vi "Climb_Set.vi"   [LabVIEW 2019]
uses:
  Globals/Climb_Globals.vi
types:
  T1 = enum16{"No-Op", "Extending", "Clamping", "Balancing", "Manual_Control"}
  T2 = typedef "Climb_Cluster.ctl" = cluster{"Control_State":T3, "Extend_Climber?":bool, "Clamp?":bool, "Balance?":bool, "Transverse_Throttle":dbl, "Elevator_Throttle":dbl, "Control_Panel_Setpoint?":bool, "Auto-Balance":bool, "Pivot_Throttle":dbl}
  T3 = typedef "Climb_States.ctl" = enum16{"No-Op", "Extending", "Clamping", "Balancing", "Manual_Control"}
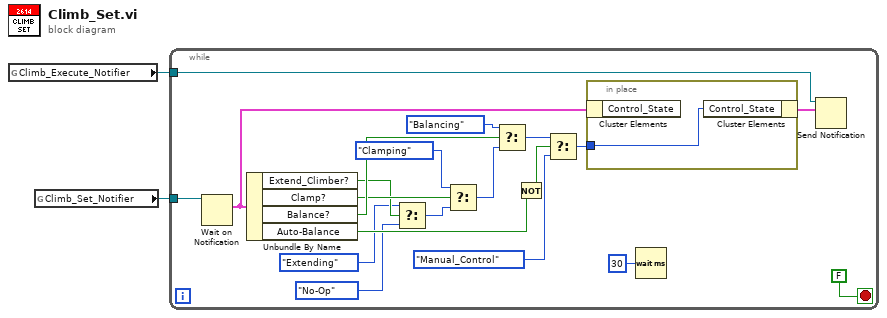
[diagram p0: block diagram]
diagram:
  n1 = global read "Climb_Globals.vi" "Climb_Execute_Notifier"() -> (w1:refnum<notifier>)
  n2 = global read "Climb_Globals.vi" "Climb_Set_Notifier"() -> (w2:refnum<notifier>)
  n3 = while {
    tunnel: w2 -> [w22]
    tunnel: w1 -> [w21]
    stop <- FALSE stop-if-true
    n4 = Wait on Notification(notifier=w22) -> (notification=w19:T2)  [unwired: 3 in, 3 out]
    n5 = Unbundle By Name(w19) -> ("Extend_Climber?"=w13:bool, "Clamp?"=w14:bool, "Balance?"=w16:bool, "Auto-Balance"=w18:bool)
    n6 = Select(t=T1."Extending" ("Control_State"), s=w13, f=T1."No-Op" ("Control_State")) -> (s? t:f=w12:T1)
    n7 = Select(t=T1."Clamping" ("Control_State"), s=w14, f=w12) -> (s? t:f=w15:T1)
    n8 = Select(t=T1."Balancing" ("Control_State"), s=w16, f=w15) -> (s? t:f=w17:T1)
    n9 = Not(x=w18) -> (.not. x?=w4:bool)
    n10 = Select(t=w17, s=w4, f=T1."Manual_Control" ("Control_State")) -> (s? t:f=w11:T1)
    n11 = in-place {
      in-place-border: w11 -> [w23]
      n12 = in-place-cluster #1(w19) -> ()  [unwired: 1 out]
      n13 = in-place-cluster #1("Control_State"=w23) -> (w10:T2)
    }
    n14 = Wait (ms)(milliseconds to wait=u32 30) -> ()  [unwired: 1 out]
    n15 = Send Notification(notification=w10, notifier=w21) -> ()  [unwired: 1 in, 2 out]
  }
